vi "getCriticalError.vi"(8 "ErrorIn":errorcluster, 11 "QueuesIn":T1) -> (0 "ErrorOut":errorcluster, 3 "QueuesOut":T1)   [LabVIEW 2019]
uses:
  utilities/Queues.ctl
  UIVIs/UIInput.ctl
  UIVIs/UIOutput.ctl
  UIVIs/AccelerationDataFrames.ctl
  communicateWebServicesVIs/WebServicesData.ctl
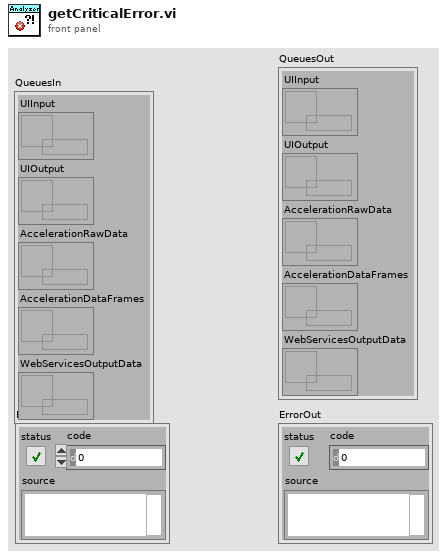
[diagram p1: front panel]
types:
  T1 = typedef "Queues.ctl" = cluster{"UIInput":refnum<queue>, "UIOutput":refnum<queue>, "AccelerationRawData":refnum<queue>, "AccelerationDataFrames":refnum<queue>, "WebServicesOutputData":refnum<queue>}
  T2 = typedef "UIOutput.ctl" = cluster{"Aquiring data":bool, "CriticalError":errorcluster, "InternalError":errorcluster, "FIFO overflow":bool, "Analyzing data":bool}
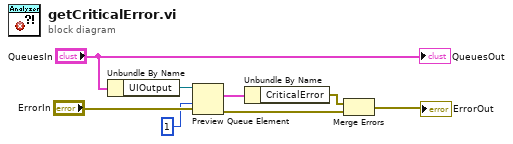
[diagram p0: block diagram]
diagram:
  n1 = Unbundle By Name("QueuesIn") -> ("UIOutput"=w8:refnum<queue>)
  n2 = Preview Queue Element(queue=w8, timeout in ms (-1)=1, error in (no error)="ErrorIn") -> (element=w5:T2, error out=w3:errorcluster)  [unwired: 2 out]
  n3 = Unbundle By Name(w5) -> ("CriticalError"=w4:errorcluster)
  n4 = Merge Errors(w4, w3) -> (→"ErrorOut":errorcluster)
  "QueuesOut" <- "QueuesIn"
